vi "display_michelle_PTK_visjitter_stopadded_RandCont_PsuedoCO_TSLogV2.vi"() -> ()   [LabVIEW 2019]
uses:
  <vilib>/Analysis/Matrix/Datatypes/RealMatrix.ctl
  <vilib>/Utility/file.llb/Write Delimited Spreadsheet (DBL).vi
  <vilib>/Analysis/Matrix/NI_Matrix.lvlib
panel:
  out "lambda":dbl
  out "maxITI":dbl
  out "minITI":dbl
  out "goEXP":dbl
  out "meanITI":dbl
  out "Lag1":dbl
  out "TSLog":dbl[][](array[numeric])
  out "TSLog2":dbl[][](array[numeric])
  out "Initialtime":dbl
  out "TSLog1":dbl[][](array[numeric])
  out "ArrayTemp3":T1
  out "StimID2":dbl
  out "Contrast":dbl
  out "TimeOutCounter":i32
  out "ElapsedTime_M":dbl
  out "Base_Contrast":dbl
  out "CurrentTrial":u32=1
  out "Jitter":dbl
  out "BaseITI":dbl
  out "VisStimDuration":dbl
  in  "Stop":bool
  out "Num trials":u32=204
  out "ISI Time":dbl
  out "Stim TS":dbl
  out "Output":dbl[][](array[numeric])
  out "Output frame":T1
  out "Array temp1":T1
  out "Elapsed Time":dbl
  out "Display":bool=TRUE
  out "Trial":u32=1
  out "reward":dbl[](array[numeric])
  out "stim_id":dbl[](array[numeric])
  out "stim_loaded":dbl
  out "Timings":dbl[](array[numeric])
  out "Stimuli Loaded?":bool
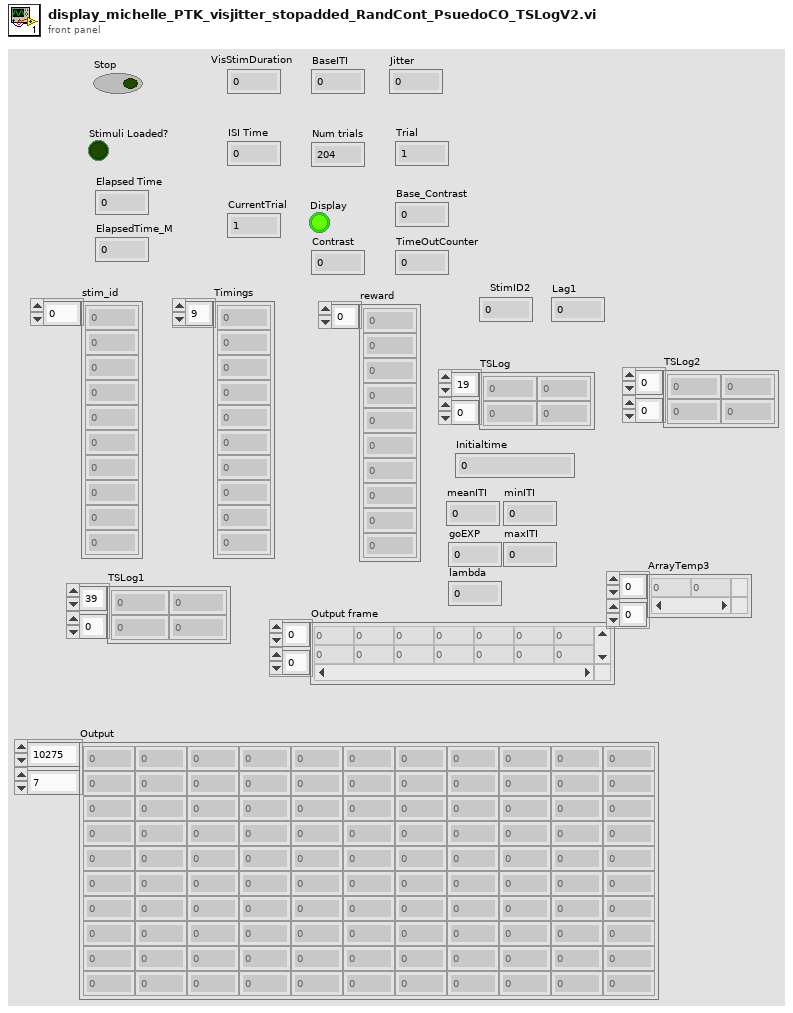
[diagram p1: front panel]
types:
  T1 = typedef "NI_Matrix.lvlib/RealMatrix.ctl" = dbl[][]
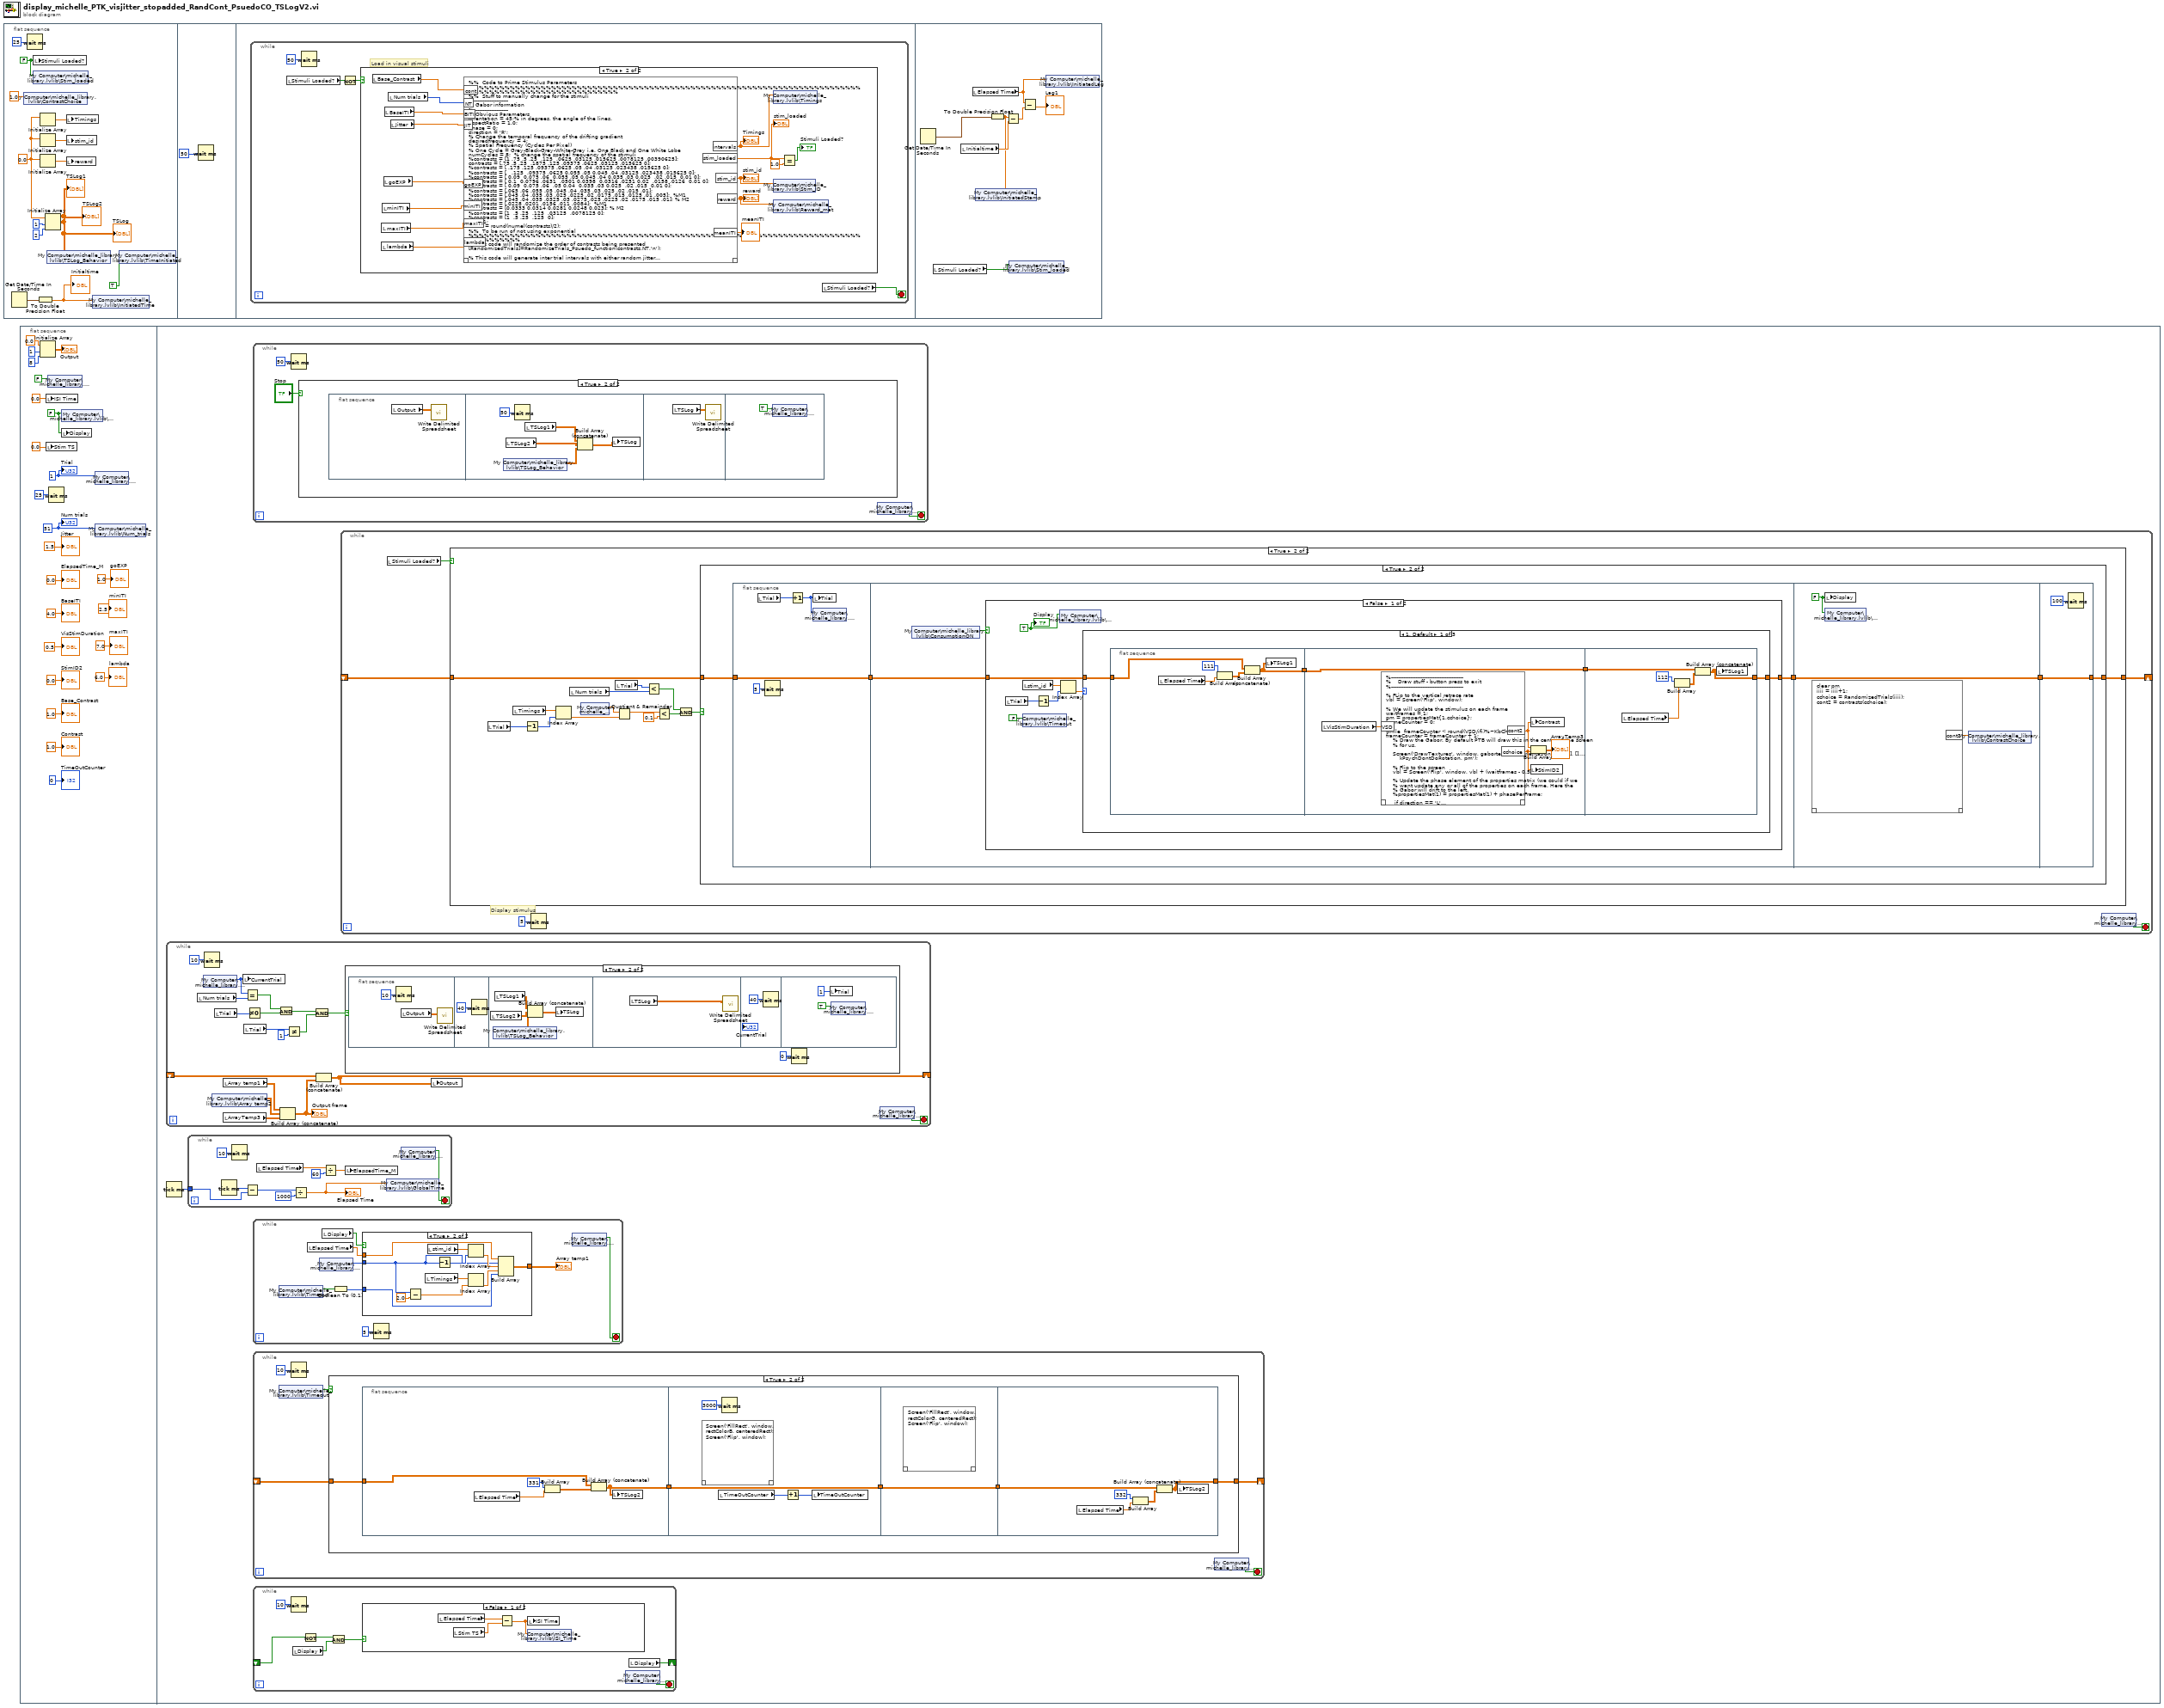
[diagram p0: block diagram]
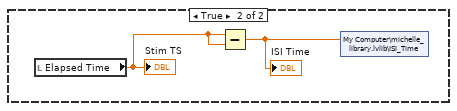
[diagram p5: hidden frame]
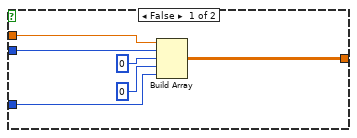
[diagram p6: hidden frame]
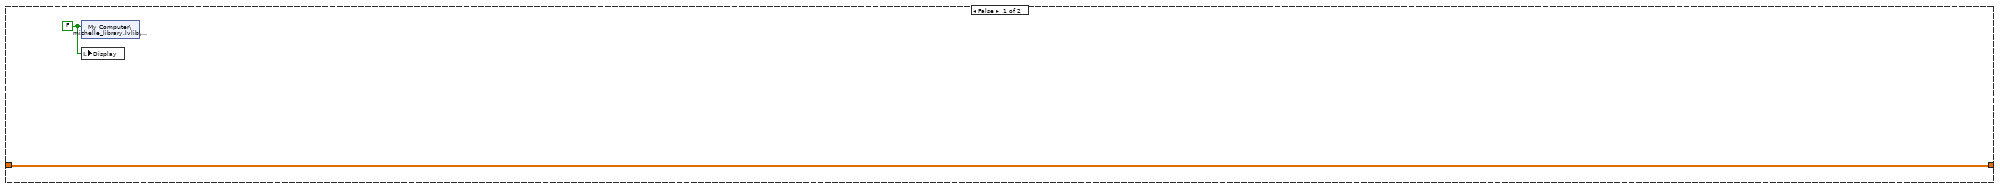
[diagram p9: hidden frame]
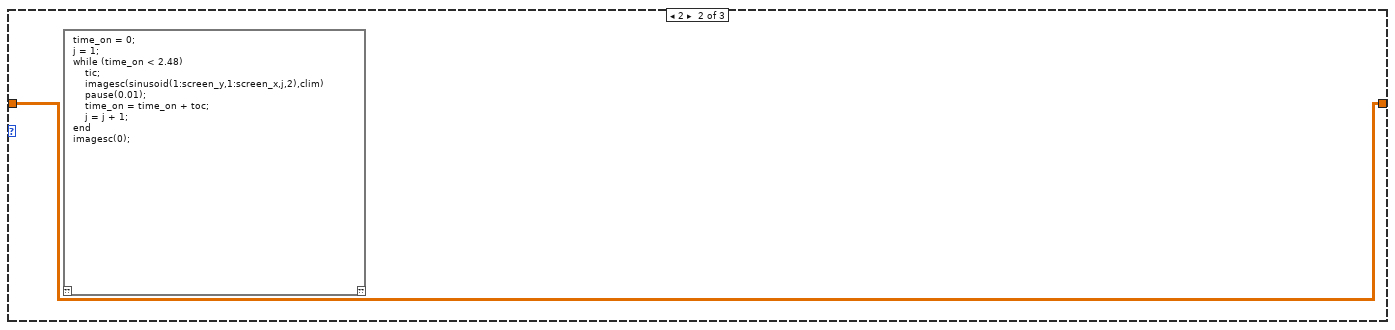
[diagram p10: hidden frame]
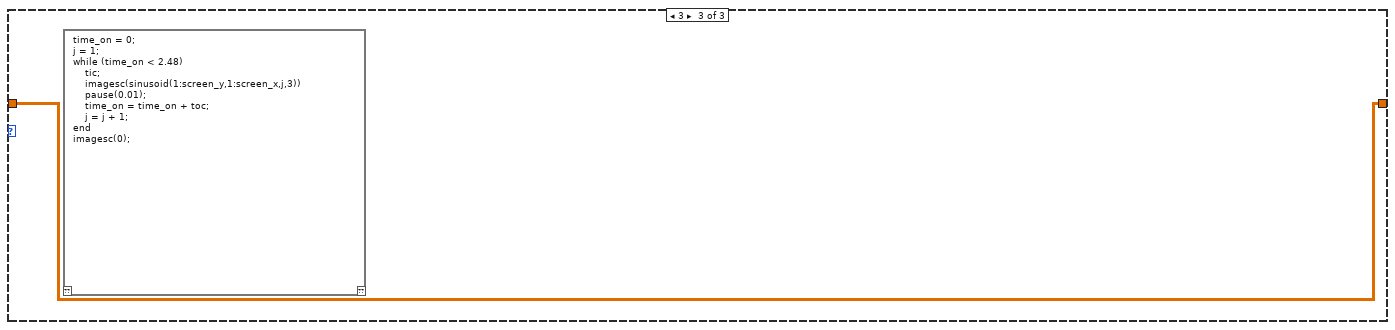
[diagram p11: hidden frame]
diagram:
  n1 = flat-sequence {
    frame #0 {
      w7 = 0.0 ("element")
      w9 = FALSE ("Stimuli Loaded?")
      n2 = Get Date/Time In Seconds() -> (seconds since 1Jan1904=w4:timestamp)
      n3 = shared-variable "My Computer\\michelle_library.lvlib\\ContrastChoice"(1.0) -> ()  [unwired: 1 in, 1 out]
      n4 = Wait (ms)(milliseconds to wait=u32 25) -> ()  [unwired: 1 out]
      n5 = local write "Stimuli Loaded?"(w9) -> ()
      n6 = shared-variable "My Computer\\michelle_library.lvlib\\Stim_loaded"(w9) -> ()  [unwired: 1 in, 1 out]
      n7 = To Double Precision Float(number=w4) -> (double precision float=w3:dbl)
      "Initialtime" <- w3
      n8 = Initialize Array(w7) -> (w12:dbl[])  [unwired: 1 in]
      n9 = Initialize Array(w7) -> (w11:dbl[])  [unwired: 1 in]
      n10 = Initialize Array(w7) -> (w10:dbl[])  [unwired: 1 in]
      n11 = Initialize Array(w7, 1, 2) -> (w1:dbl[][])
      "TSLog1" <- w1
      "TSLog2" <- w1
      "TSLog" <- w1
      n12 = shared-variable "My Computer\\michelle_library.lvlib\\TSLog_Behavior"(w1) -> ()  [unwired: 1 in, 1 out]
      n13 = local write "Timings"(w12) -> ()
      n14 = local write "stim_id"(w11) -> ()
      n15 = local write "reward"(w10) -> ()
      n16 = shared-variable "My Computer\\michelle_library.lvlib\\InitiatedTime"(w3) -> ()  [unwired: 1 in, 1 out]
      n17 = shared-variable "My Computer\\michelle_library.lvlib\\TimeInitiated"(TRUE) -> ()  [unwired: 1 in, 1 out]
    }
    frame #1 {
      n18 = Wait (ms)(milliseconds to wait=u32 50) -> ()  [unwired: 1 out]
    }
    frame #2 {
      n19 = while {
        stop <- w15 stop-if-true
        # "Load in visual stimuli"
        n20 = local read "Stimuli Loaded?"() -> (w17:bool)
        n21 = Wait (ms)(milliseconds to wait=u32 50) -> ()  [unwired: 1 out]
        n22 = Not(x=w17) -> (.not. x?=w16:bool)
        n23 = case shown="True" w16 {
          frame False {
          }
          frame True {
            n24 = local read "Base_Contrast"() -> (w25:dbl)
            n25 = local read "maxITI"() -> (w21:dbl)
            n26 = local read "lambda"() -> (w22:dbl)
            n27 = local read "minITI"() -> (w20:dbl)
            n28 = local read "goEXP"() -> (w19:dbl)
            n29 = local read "BaseITI"() -> (w27:dbl)
            n30 = local read "Num trials"() -> (w28:u32)
            n31 = local read "Jitter"() -> (w26:dbl)
            n32 = script code="%%  Code to Prime Stimulus Parameters\n%%%%%%%%%%%%%%%%%%%%%%%%%%%%%%%%%%%%%%%%%%%%%%%%%%%%%%%%%%%%%%%%%%%%%%%%%%%%%%%%%%%%%%%%%%%%%%%%%%%%%%%%%\n%%  Stuff to manually change for the stimuli\n%--------------------\n% Gabor information\n%--------------------\n% Obvious Parameters\norientation = 45;% in degrees, the angle of the lines.\naspectRatio = 1.0;\nphase = 0;\ndirection = 'R';\n% Change the temporal frequency of the drifting gradient\ndesiredfrequency = 4;\n% Spatial Frequency (Cycles Per Pixel)\n% One Cycle = Grey-Black-Grey-White-Grey i.e. One Black and One White Lobe\nnumCycles = 8;  % change the spatial frequency of the stimuli\n%contrasts = [1 .75 .5 .25  .125  .0625 .03125 .015625 .0078125 .00390625];\ncontrasts = [.75 .5 .25  .1875 .125 .09375 .0625 .03125 .015625 0];\n%contrasts = [ .175 .125 .09375 .0625 .05 .04 .03125 .023438 .015625 0];\n%contrasts = [   .125  .09375 .0625 0.055 .05 0.045 .04 .03125 .023438 .015625 0];\n%contrasts = [ 0.09  0.075 .06  0.055 .05 0.045 .04 0.035 .03 0.025  .02 .015  0.01 0];\n%contrasts = [ 0.1  0.0796 .0631  .0501 0.0398  0.0316 .0251 0.02  .0158 .0126  0.01 0];\n%contrasts = [ 0.09  0.075 .06  .05 0.04  0.035 .03 0.025  .02 .015  0.01 0];\n%contrasts = [.065 .06 .055 .05 .045 .04 .035 .03 .025 .02 .015 .01];\n%contrasts = [.045 .04 .035 .03 .025 .0225 .02 .0175 .015 .0125 .01 .005];  %M1\n%contrasts = [.045 .04 .035 .0325 .03 .0275 .025 .0225 .02 .0175 .015 .01]; % M2\n%contrasts = [.0228 .0201 .0156 .011 .0084];  %M1\n%contrasts = [0.0333 0.0314 0.0281 0.0248 0.023]; % M2\n%contrasts = [1  .5 .25  .125  .03125  .0078125 0];\n%contrasts = [1  .5 .25  .125  0];\ngo = 1;\nmaxc = round(numel(contrasts)/2);\n%%  To be run of not using exponential\n%%%%%%%%%%%%%%%%%%%%%%%%%%%%%%%%%%%%%%%%%%%%%%%%%%%%%%%%%%%%%%%%%%%%%%%%%%%%%%%%%%%%%%\n% This code will randomize the order of contrasts being presented\n[RandomizedTrials]=RandomizeTrials_Psuedo_function(contrasts,NT,'n');\n\n% This code will generate inter trial intervals with either random jitter\n% or based on an exponential distribution\nif goEXP < 1\n     jit = JIT;\n     jitter = rand(1,NT);\n     jitter = 2*jit*(jitter- .5);\n     ITIbase = BITI;\n     intervals = [ones(1,NT)*ITIbase];\n     intervals = intervals + jitter;\nelseif goEXP > 0\n     intervals = exponentialITI(1/lambda, minITI, maxITI, NT);\nend\n\n%%  Prep the stimulus presentation software\n%%%%%%%%%%%%%%%%%%%%%%%%%%%%%%%%%%%%%%%%%%%%%%%%%%%%%%%%%%%%%%%%%%%%%%%%%%%\nsca;\nclose all;\n% Setup PTB with some default values\nPsychDefaultSetup(2);\n% Set the screen number to the external secondary monitor if there is one connected\nscreenNumber = max(Screen('Screens'));\n\n% Define black, white and grey\nwhite = WhiteIndex(screenNumber);\nblack = BlackIndex(screenNumber);\ngrey = white / 2;\n\n% Open the screen & define it's dimensions\n[window, windowRect] = PsychImaging('OpenWindow', screenNumber, grey,...\n    [], 32, 2, [], [], kPsychNeedRetinaResolution);\n[screenXpixels, screenYpixels] = Screen('WindowSize', window);\n[xCenter, yCenter] = RectCenter(windowRect);\n\n% Get the vertical refresh rate of the monitor\nifi = Screen('GetFlipInterval', window);\n\n% Set maximum priority level\ntopPriorityLevel = MaxPriority(window);\nPriority(topPriorityLevel);\n\n\n% Build a procedural gabor texture (Note: to get a \"standard\" Gabor patch\n% we set a grey background offset, disable normalisation, and set a\n% pre-contrast multiplier of 0.5).\n% Dimension of the region where will draw the Gabor in pixels\ngaborDimPix = windowRect(3);\n% Sigma of Gaussian  (how much to fade around the edges)\nsigma = gaborDimPix / 0;  % change the 0 value to alter the fading\nphasePerFrame = desiredfrequency*360*ifi;\nfreq = numCycles / gaborDimPix;\n\nbackgroundOffset = [0.5 0.5 0.5 0.0];\ndisableNorm = 1;\npreContrastMultiplier = 0.5;\ngabortex = CreateProceduralGabor(window, gaborDimPix, gaborDimPix, [],...\n    backgroundOffset, disableNorm, preContrastMultiplier);\n\n% Randomise the phase of the Gabors and make a properties matrix.\nfor N = 1:numel(contrasts)\npropertiesMat{1,N} = [phase, freq, sigma, contrasts(N), aspectRatio, 0, 0, 0];\nend\n\niiii = 1;\ncchoice = RandomizedTrials(iiii);\ncont2 = contrasts(cchoice);\npm = propertiesMat{1,1};\n\n\n%%  Build up the rectangles for the pause and hold screen\nbaseRect = [0 0 screenXpixels screenYpixels];\ncenteredRect = CenterRectOnPointd(baseRect, xCenter, yCenter);\nrectColorB = [0 0 0];\nrectColorG = [128 128 128]/255;\n\n%%  Finalize the trial data and orders\nstim_id = [ones(1,NT)*1];\nreward = [ones(1,NT)*1];\nmeanITI = nanmean(intervals);\nrand_idx1 = randperm(NT);\nrand_idx2 = randperm(NT);\nintervals = intervals(rand_idx2);\nstim_id = stim_id(rand_idx2);\nreward = reward(rand_idx2);\n%%  All Done!\n%  indicate that the necessary preloading of data has been completed.\nstim_loaded = 1;" ("Script Node")("NT"=w28, "BITI"=w27, "JIT"=w26, "cont"=w25, "goEXP"=w19, "minITI"=w20, "maxITI"=w21, "lambda"=w22) -> ("stim_loaded"=w33:dbl, "intervals"=w29:dbl[], "stim_id"=w30:dbl[], "reward"=w31:dbl[], "meanITI"=→"meanITI":dbl)  [unwired: 1 in, 1 out]
            "stim_loaded" <- w33
            "Timings" <- w29
            "stim_id" <- w30
            "reward" <- w31
            n33 = shared-variable "My Computer\\michelle_library.lvlib\\Timings"(w29) -> ()  [unwired: 1 in, 1 out]
            n34 = shared-variable "My Computer\\michelle_library.lvlib\\Stim_ID"(w30) -> ()  [unwired: 1 in, 1 out]
            n35 = shared-variable "My Computer\\michelle_library.lvlib\\Reward_mat"(w31) -> ()  [unwired: 1 in, 1 out]
            n36 = Equal?(x=w33, y=1.0) -> (x = y?=→"Stimuli Loaded?":bool)
          }
        }
        n37 = local read "Stimuli Loaded?"() -> (w15:bool)
      }
    }
    frame #3 {
      n38 = Get Date/Time In Seconds() -> (seconds since 1Jan1904=w40:timestamp)
      n39 = local read "Stimuli Loaded?"() -> (w35:bool)
      n40 = local read "Initialtime"() -> (w39:dbl)
      n41 = local read "Elapsed Time"() -> (w34:dbl)
      n42 = To Double Precision Float(number=w40) -> (double precision float=w37:dbl)
      n43 = shared-variable "My Computer\\michelle_library.lvlib\\InitiatedStamp"(w37) -> ()  [unwired: 1 in, 1 out]
      n44 = Subtract(x=w37, y=w39) -> (x-y=w38:dbl)
      n45 = shared-variable "My Computer\\michelle_library.lvlib\\Stim_loaded"(w35) -> ()  [unwired: 1 in, 1 out]
      n46 = Subtract(x=w34, y=w38) -> (x-y=→"Lag1":dbl)
      n47 = shared-variable "My Computer\\michelle_library.lvlib\\InitiatedLag"(w34) -> ()  [unwired: 1 in, 1 out]
    }
  }
  n48 = flat-sequence {
    frame #0 {
      w55 = u32 51
      w61 = FALSE ("Display")
      w63 = u32 1 ("Trial")
      n49 = Initialize Array(0.0 ("element"), 1 ("dimension size"), 8 ("dimension size")) -> (→"Output":dbl[][])
      n50 = local write "ISI Time"(0.0 ("ISI Time")) -> ()
      n51 = local write "Stim TS"(0.0 ("Stim TS")) -> ()
      n52 = shared-variable "My Computer\\michelle_library.lvlib\\Stop"(FALSE ("Stop")) -> ()  [unwired: 1 in, 1 out]
      n53 = Wait (ms)(milliseconds to wait=u32 25) -> ()  [unwired: 1 out]
      n54 = shared-variable "My Computer\\michelle_library.lvlib\\Display"(w61) -> ()  [unwired: 1 in, 1 out]
      n55 = local write "Display"(w61) -> ()
      n56 = shared-variable "My Computer\\michelle_library.lvlib\\Trial"(w63) -> ()  [unwired: 1 in, 1 out]
      n57 = shared-variable "My Computer\\michelle_library.lvlib\\Num_trials"(w55) -> ()  [unwired: 1 in, 1 out]
      "Trial" <- w63
      "Num trials" <- w55
      "VisStimDuration" <- 0.5
      "BaseITI" <- 4.0
      "Jitter" <- 1.5
      "Base_Contrast" <- 1.0
      "ElapsedTime_M" <- 0.0
      "TimeOutCounter" <- 0
      "Contrast" <- 1.0
      "StimID2" <- 0.0
      "goEXP" <- 1.0
      "minITI" <- 2.5
      "maxITI" <- 7.0
      "lambda" <- 6.0
    }
    frame #1 {
      n58 = while {
        shift-right: [w163] -> _
        shift-left: _ -> [w164]
        stop <- w166 stop-if-true
        n59 = local read "Num trials"() -> (w159:u32)
        n60 = shared-variable "My Computer\\michelle_library.lvlib\\Trial"() -> (w150:u32)  [unwired: 1 in, 1 out]
        n61 = Wait (ms)(milliseconds to wait=u32 10) -> ()  [unwired: 1 out]
        n62 = shared-variable "My Computer\\michelle_library.lvlib\\Array temp2"() -> (w161:dbl[][])  [unwired: 1 in, 1 out]
        n63 = local read "Trial"() -> (w157:u32)
        n64 = local read "Array temp1"() -> (w162:T1)
        n65 = local read "ArrayTemp3"() -> (w149:T1)
        n66 = local write "CurrentTrial"(w150) -> ()
        n67 = local read "Trial"() -> (w156:u32)
        n68 = Equal?(x=w150, y=w159) -> (x = y?=w158:bool)
        n69 = Not Equal To 0?(x=w157) -> (x != 0?=w153:bool)
        n70 = And(x=w158, y=w153) -> (x .and. y?=w151:bool)
        n71 = Build Array (concatenate)(w162, w161, w149) -> (w160:T1)
        "Output frame" <- w160
        n72 = Not Equal?(x=w156, y=1) -> (x != y?=w155:bool)
        n73 = And(x=w151, y=w155) -> (x .and. y?=w152:bool)
        n74 = Build Array (concatenate) ("Build Matrix")(w164, w160) -> (w163:T1)
        n75 = case shown="True" w152 {
          frame False {
          }
          frame True {
            n76 = flat-sequence {
              frame #0 {
                n77 = Wait (ms)(milliseconds to wait=u32 10) -> ()  [unwired: 1 out]
                n78 = local read "Output"() -> (w169:dbl[][])
                n79 = call-poly <vilib>:"Write Delimited Spreadsheet.vi"("2D data"=w169) -> ()  [unwired: 13 in, 2 out]
              }
              frame #1 {
                n80 = Wait (ms)(milliseconds to wait=u32 40) -> ()  [unwired: 1 out]
              }
              frame #2 {
                n81 = local read "TSLog2"() -> (w174:dbl[][])
                n82 = shared-variable "My Computer\\michelle_library.lvlib\\TSLog_Behavior"() -> (w172:dbl[][])  [unwired: 1 in, 1 out]
                n83 = local read "TSLog1"() -> (w173:dbl[][])
                n84 = Build Array (concatenate) ("Build Matrix")(w173, w174, w172) -> (w171:T1)
                n85 = local write "TSLog"(w171) -> ()
              }
              frame #3 {
                n86 = local read "TSLog"() -> (w175:dbl[][])
                n87 = call-poly <vilib>:"Write Delimited Spreadsheet.vi"("2D data"=w175) -> ()  [unwired: 13 in, 2 out]
              }
              frame #4 {
                n88 = Wait (ms)(milliseconds to wait=u32 40) -> ()  [unwired: 1 out]
              }
              frame #5 {
                n89 = local write "Trial"(1) -> ()
                n90 = shared-variable "My Computer\\michelle_library.lvlib\\Stop"(TRUE) -> ()  [unwired: 1 in, 1 out]
              }
            }
            n91 = Wait (ms)(milliseconds to wait=0) -> ()  [unwired: 1 out]
          }
        }
        n92 = local write "Output"(w163) -> ()
        n93 = shared-variable "My Computer\\michelle_library.lvlib\\Stop"() -> (w166:bool)  [unwired: 1 in, 1 out]
      }
      n94 = Tick Count (ms)() -> (millisecond timer value=w64:u32)
      n95 = while {
        tunnel: w64 -> [w146]
        stop <- w143 stop-if-true
        n96 = Tick Count (ms)() -> (millisecond timer value=w147:u32)
        n97 = Wait (ms)(milliseconds to wait=u32 10) -> ()  [unwired: 1 out]
        n98 = Subtract(x=w147, y=w146) -> (x-y=w144:u32)
        n99 = local read "Elapsed Time"() -> (w141:dbl)
        n100 = Divide(x=w144, y=u32 1000) -> (x/y=w139:dbl)
        "Elapsed Time" <- w139
        n101 = Divide(x=w141, y=60) -> (x/y=w140:dbl)
        n102 = local write "ElapsedTime_M"(w140) -> ()
        n103 = shared-variable "My Computer\\michelle_library.lvlib\\GlobalTime"(w139) -> ()  [unwired: 1 in, 1 out]
        n104 = shared-variable "My Computer\\michelle_library.lvlib\\Stop"() -> (w143:bool)  [unwired: 1 in, 1 out]
      }
      n105 = while {
        stop <- w67 stop-if-true
        n106 = Wait (ms)(milliseconds to wait=50) -> ()  [unwired: 1 out]
        n107 = case shown="True" "Stop" {
          frame False {
          }
          frame True {
            n108 = flat-sequence {
              frame #0 {
                n109 = local read "Output"() -> (w68:dbl[][])
                n110 = call-poly <vilib>:"Write Delimited Spreadsheet.vi"("2D data"=w68) -> ()  [unwired: 13 in, 2 out]
              }
              frame #1 {
                n111 = shared-variable "My Computer\\michelle_library.lvlib\\TSLog_Behavior"() -> (w69:dbl[][])  [unwired: 1 in, 1 out]
                n112 = local read "TSLog2"() -> (w72:dbl[][])
                n113 = Wait (ms)(milliseconds to wait=50) -> ()  [unwired: 1 out]
                n114 = local read "TSLog1"() -> (w71:dbl[][])
                n115 = Build Array (concatenate) ("Build Matrix")(w71, w72, w69) -> (w70:T1)
                n116 = local write "TSLog"(w70) -> ()
              }
              frame #2 {
                n117 = local read "TSLog"() -> (w74:dbl[][])
                n118 = call-poly <vilib>:"Write Delimited Spreadsheet.vi"("2D data"=w74) -> ()  [unwired: 13 in, 2 out]
              }
              frame #3 {
                n119 = shared-variable "My Computer\\michelle_library.lvlib\\Stop"(TRUE) -> ()  [unwired: 1 in, 1 out]
              }
            }
          }
        }
        n120 = shared-variable "My Computer\\michelle_library.lvlib\\Stop"() -> (w67:bool)  [unwired: 1 in, 1 out]
      }
      n121 = while {
        stop <- w116 stop-if-true
        n122 = shared-variable "My Computer\\michelle_library.lvlib\\Timeout"() -> (w114:bool)  [unwired: 1 in, 1 out]
        n123 = local read "Elapsed Time"() -> (w120:dbl)
        n124 = shared-variable "My Computer\\michelle_library.lvlib\\Trial"() -> (w118:u32)  [unwired: 1 in, 1 out]
        n125 = local read "Display"() -> (w117:bool)
        n126 = Boolean To (0,1)(Boolean=w114) -> (0, 1=w115:i16)
        n127 = case shown="True" w117 {
          tunnel: w118 -> [w126 w129]
          tunnel: w120 -> [w127 w136]
          tunnel: [w125 w137] -> w119
          tunnel: w115 -> [w122 w131]
          frame False {
            n128 = Build Array(w127, w126, u32 0 ("milliseconds to wait"), 0, w122) -> (w125:T1)
          }
          frame True {
            n129 = Subtract(x=w129, y=2.0) -> (x-y=w128:dbl)
            n130 = local read "Timings"() -> (w134:dbl[])
            n131 = local read "stim_id"() -> (w138:dbl[])
            n132 = Decrement(x=w129) -> (x-1=w133:u32)
            n133 = Index Array(array=w138, index=w133) -> (element=w135:dbl)
            n134 = Index Array(array=w134, index=w128) -> (element=w132:dbl)
            n135 = Build Array(w136, w129, w135, w132, w131) -> (w137:T1)
          }
        }
        "Array temp1" <- w119
        n136 = Wait (ms)(milliseconds to wait=u32 5) -> ()  [unwired: 1 out]
        n137 = shared-variable "My Computer\\michelle_library.lvlib\\Stop"() -> (w116:bool)  [unwired: 1 in, 1 out]
      }
      n138 = while {
        shift-right: [w76] -> _
        shift-left: _ -> [w77]
        stop <- w80 stop-if-true
        n139 = shared-variable "My Computer\\michelle_library.lvlib\\Timeout"() -> (w78:bool)  [unwired: 1 in, 1 out]
        n140 = Wait (ms)(milliseconds to wait=u32 10) -> ()  [unwired: 1 out]
        n141 = case shown="True" w78 {
          tunnel: w77 -> [w81 w86]
          tunnel: [w81 w85] -> w76
          frame False {
          }
          frame True {
            n142 = flat-sequence {
              tunnel: w86 -> [w89]
              tunnel: [w88] -> w83
              tunnel: [w92] -> w84
              tunnel: w83 -> [w92]
              tunnel: w84 -> [w96]
              tunnel: [w96] -> w82
              tunnel: [w98] -> w85
              tunnel: w82 -> [w99]
              frame #0 {
                n143 = local read "Elapsed Time"() -> (w87:dbl)
                n144 = Build Array(331, w87) -> (w91:T1)
                n145 = Build Array (concatenate) ("Build Matrix")(w89, w91) -> (w88:T1)
                n146 = local write "TSLog2"(w88) -> ()
              }
              frame #1 {
                n147 = script code="Screen('FillRect', window, rectColorB, centeredRect);\nScreen('Flip', window);"() -> ()  [unwired: 1 in, 1 out]
                n148 = local read "TimeOutCounter"() -> (w94:i32)
                n149 = Wait (ms)(milliseconds to wait=u32 3000) -> ()  [unwired: 1 out]
                n150 = Increment(x=w94) -> (x+1=w93:i32)
                n151 = local write "TimeOutCounter"(w93) -> ()
              }
              frame #2 {
                n152 = script code="Screen('FillRect', window, rectColorG, centeredRect);\nScreen('Flip', window);"() -> ()  [unwired: 1 in, 1 out]
              }
              frame #3 {
                n153 = local read "Elapsed Time"() -> (w97:dbl)
                n154 = Build Array(332, w97) -> (w100:T1)
                n155 = Build Array (concatenate) ("Build Matrix")(w99, w100) -> (w98:T1)
                n156 = local write "TSLog2"(w98) -> ()
              }
            }
          }
        }
        n157 = shared-variable "My Computer\\michelle_library.lvlib\\Stop"() -> (w80:bool)  [unwired: 1 in, 1 out]
      }
      n158 = while {
        shift-right: [w106] -> _
        shift-left: _ -> [w105]
        stop <- w108 stop-if-true
        n159 = Wait (ms)(milliseconds to wait=u32 10) -> ()  [unwired: 1 out]
        n160 = local read "Display"() -> (w103:bool)
        n161 = Not(x=w105) -> (.not. x?=w104:bool)
        n162 = And(x=w104, y=w103) -> (x .and. y?=w102:bool)
        n163 = case shown="False" w102 {
          frame False {
            n164 = local read "Elapsed Time"() -> (w109:dbl)
            n165 = local read "Stim TS"() -> (w111:dbl)
            n166 = Subtract(x=w109, y=w111) -> (x-y=w110:dbl)
            n167 = local write "ISI Time"(w110) -> ()
            n168 = shared-variable "My Computer\\michelle_library.lvlib\\ISI_Time"(w110) -> ()  [unwired: 1 in, 1 out]
          }
          frame True {
            n169 = local read "Elapsed Time"() -> (w112:dbl)
            "Stim TS" <- w112
            n170 = Subtract(x=w112, y=w112) -> (x-y=w113:dbl)
            "ISI Time" <- w113
            n171 = shared-variable "My Computer\\michelle_library.lvlib\\ISI_Time"(w113) -> ()  [unwired: 1 in, 1 out]
          }
        }
        n172 = shared-variable "My Computer\\michelle_library.lvlib\\Stop"() -> (w108:bool)  [unwired: 1 in, 1 out]
        n173 = local read "Display"() -> (w106:bool)
      }
      n174 = while {
        shift-right: [w179] -> _
        shift-left: _ -> [w180]
        stop <- w182 stop-if-true
        # "Display stimulus"
        n175 = local read "Stimuli Loaded?"() -> (w181:bool)
        n176 = case shown="True" w181 {
          tunnel: w180 -> [w184 w186]
          tunnel: [w184 w185] -> w179
          frame False {
          }
          frame True {
            n177 = local read "Trial"() -> (w187:u32)
            n178 = local read "Timings"() -> (w196:dbl[])
            n179 = Decrement(x=w187) -> (x-1=w188:u32)
            n180 = Index Array(array=w196, index=w188) -> (element=w195:dbl)
            n181 = local read "Num trials"() -> (w191:u32)
            n182 = shared-variable "My Computer\\michelle_library.lvlib\\ISI"() -> (w190:dbl)  [unwired: 1 in, 1 out]
            n183 = local read "Trial"() -> (w194:u32)
            n184 = Quotient & Remainder(x=w190, y=w195) -> (x-y*floor(x/y)=w198:dbl)  [unwired: 1 out]
            n185 = Less?(x=w194, y=w191) -> (x < y?=w193:bool)
            n186 = Less?(x=w198, y=0.1) -> (x < y?=w192:bool)
            n187 = And(x=w193, y=w192) -> (x .and. y?=w189:bool)
            n188 = case shown="True" w189 {
              tunnel: w186 -> [w199 w204]
              tunnel: [w199 w203] -> w185
              frame False {
                w200 = FALSE ("Display")
                n189 = shared-variable "My Computer\\michelle_library.lvlib\\Display"(w200) -> ()  [unwired: 1 in, 1 out]
                n190 = local write "Display"(w200) -> ()
              }
              frame True {
                n191 = flat-sequence {
                  tunnel: [w206] -> w205
                  tunnel: w204 -> [w206]
                  tunnel: w205 -> [w211]
                  tunnel: [w210] -> w201
                  tunnel: [w243] -> w202
                  tunnel: w201 -> [w243]
                  tunnel: [w246] -> w203
                  tunnel: w202 -> [w246]
                  frame #0 {
                    n192 = local read "Trial"() -> (w209:u32)
                    n193 = Wait (ms)(milliseconds to wait=u32 5) -> ()  [unwired: 1 out]
                    n194 = Increment(x=w209) -> (x+1=w208:u32)
                    n195 = local write "Trial"(w208) -> ()
                    n196 = shared-variable "My Computer\\michelle_library.lvlib\\Trial"(w208) -> ()  [unwired: 1 in, 1 out]
                  }
                  frame #1 {
                    n197 = shared-variable "My Computer\\michelle_library.lvlib\\ConsumptionON"() -> (w212:bool)  [unwired: 1 in, 1 out]
                    n198 = case shown="False" w212 {
                      tunnel: w211 -> [w214 w242]
                      tunnel: [w213 w242] -> w210
                      frame False {
                        w215 = TRUE ("Boolean")
                        n199 = local read "Trial"() -> (w218:u32)
                        n200 = shared-variable "My Computer\\michelle_library.lvlib\\Timeout"(FALSE) -> ()  [unwired: 1 in, 1 out]
                        n201 = local read "stim_id"() -> (w220:dbl[])
                        n202 = Decrement(x=w218) -> (x-1=w217:u32)
                        n203 = shared-variable "My Computer\\michelle_library.lvlib\\Display"(w215) -> ()  [unwired: 1 in, 1 out]
                        n204 = Index Array(array=w220, index=w217) -> (element=w219:dbl)
                        n205 = case shown="1, Default" w219 {
                          tunnel: w214 -> [w224 w240 w241]
                          tunnel: [w223 w240 w241] -> w213
                          frame 1, Default {
                            n206 = flat-sequence {
                              tunnel: w224 -> [w228]
                              tunnel: [w227] -> w222
                              tunnel: w222 -> [w230]
                              tunnel: [w230] -> w221
                              tunnel: [w238] -> w223
                              tunnel: w221 -> [w237]
                              frame #0 {
                                n207 = local read "Elapsed Time"() -> (w225:dbl)
                                n208 = Build Array(111, w225) -> (w226:T1)
                                n209 = Build Array (concatenate) ("Build Matrix")(w228, w226) -> (w227:T1)
                                n210 = local write "TSLog1"(w227) -> ()
                              }
                              frame #1 {
                                n211 = local read "VisStimDuration"() -> (w232:dbl)
                                n212 = script code="%------------------------------------------\n%    Draw stuff - button press to exit\n%------------------------------------------\n\n% FLip to the vertical retrace rate\nvbl = Screen('Flip', window);\n\n% We will update the stimulus on each frame\nwaitframes = 1;\npm = propertiesMat{1,cchoice};\nframeCounter = 0;\ntic\nwhile  frameCounter < round(VSD/ifi)%~KbCheck\nframeCounter = frameCounter + 1;\n    % Draw the Gabor. By default PTB will draw this in the center of the screen\n    % for us.\n   \n    Screen('DrawTextures', window, gabortex, [], [], orientation, [], [], [], [],...\n        kPsychDontDoRotation, pm');\n\n    % Flip to the screen\n    vbl = Screen('Flip', window, vbl + (waitframes - 0.5) * ifi);\n\n    % Update the phase element of the properties matrix (we could if we\n    % want update any or all of the properties on each frame. Here the\n    % Gabor will drift to the left.\n    %propertiesMat(1) = propertiesMat(1) + phasePerFrame;\n \n     if direction == 'L'\n          pm(1) = pm(1) + phasePerFrame;\n     elseif direction =='R'\n          pm(1) = pm(1) - phasePerFrame;\n     end\n\nend\nTime(N) = toc;\nvbl = Screen('Flip', window);"("VSD"=w232) -> ("cont2"=w234:dbl, "cchoice"=w233:dbl)  [unwired: 1 in, 1 out]
                                n213 = local write "Contrast"(w234) -> ()
                                n214 = Build Array(w234, w233) -> (→"ArrayTemp3":T1)
                                n215 = local write "StimID2"(w233) -> ()
                              }
                              frame #2 {
                                n216 = local read "Elapsed Time"() -> (w235:dbl)
                                n217 = Build Array(112, w235) -> (w239:T1)
                                n218 = Build Array (concatenate) ("Build Matrix")(w237, w239) -> (w238:T1)
                                n219 = local write "TSLog1"(w238) -> ()
                              }
                            }
                          }
                          frame 2 {
                            n220 = script code="time_on = 0;\nj = 1;\nwhile (time_on < 2.48)\n    tic;\n    imagesc(sinusoid(1:screen_y,1:screen_x,j,2),clim)\n    pause(0.01);\n    time_on = time_on + toc;\n    j = j + 1;\nend\nimagesc(0);"() -> ()  [unwired: 1 in, 1 out]
                          }
                          frame 3 {
                            n221 = script code="time_on = 0;\nj = 1;\nwhile (time_on < 2.48)\n    tic;\n    imagesc(sinusoid(1:screen_y,1:screen_x,j,3))\n    pause(0.01);\n    time_on = time_on + toc;\n    j = j + 1;\nend\nimagesc(0);"() -> ()  [unwired: 1 in, 1 out]
                          }
                        }
                        "Display" <- w215
                      }
                      frame True {
                      }
                    }
                  }
                  frame #2 {
                    w245 = FALSE ("Display")
                    n222 = script code="clear pm\niiii = iiii+1;\ncchoice = RandomizedTrials(iiii);\ncont2 = contrasts(cchoice);"() -> ("cont2"=w244:dbl)  [unwired: 1 in, 1 out]
                    n223 = local write "Display"(w245) -> ()
                    n224 = shared-variable "My Computer\\michelle_library.lvlib\\Display"(w245) -> ()  [unwired: 1 in, 1 out]
                    n225 = shared-variable "My Computer\\michelle_library.lvlib\\ContrastChoice"(w244) -> ()  [unwired: 1 in, 1 out]
                  }
                  frame #3 {
                    n226 = Wait (ms)(milliseconds to wait=u32 100) -> ()  [unwired: 1 out]
                  }
                }
              }
            }
          }
        }
        n227 = Wait (ms)(milliseconds to wait=u32 5) -> ()  [unwired: 1 out]
        n228 = shared-variable "My Computer\\michelle_library.lvlib\\Stop"() -> (w182:bool)  [unwired: 1 in, 1 out]
      }
    }
  }
